vi "ConstructorEvent.vi"() -> (3 "Data Value Reference out":refnum<data-value>)   [LabVIEW 2014]
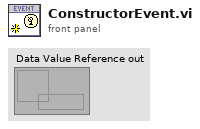
[diagram p1: front panel]
types:
  T1 = cluster{"CmdMsg":cluster{"msg":string, "data":variant}, "EQ_Name":string, "user event out":refnum<user-event>}[]
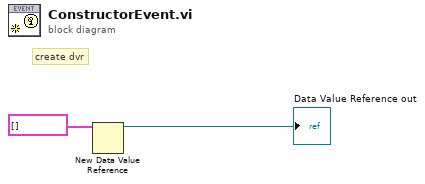
[diagram p0: block diagram]
diagram:
  # "create dvr"
  n1 = New Data Value Reference(data value=T1 []) -> (data value reference=→"Data Value Reference out":refnum<data-value>)  [unwired: 1 in, 1 out]
